vi "Set External Tn.vi"(6 "parseError? T:Yes":bool=TRUE, 8 "error in (no error)":errorcluster, 10 "Tn (3s)":u16=3 min=3 max=9999, 11 "VISA resource name":refnum<visa-resource-name>) -> (0 "error out":errorcluster, 3 "VISA resource name out":refnum<visa-resource-name>)   [LabVIEW 2015, in "JULABO DeviceDriver.lvlib"]
doc: "This VI adjusts the Resetting time <B>Tn</B> (Integral component) in case of external temperature control.\n\nCompensation of the remaining control deviation due to proportional control. An insufficient resetting time may cause instabilities to occur. An excessive resetting time will unnecessarily prolong compensation of the control difference.\nAdjustable range: <B>3 ... 9999</B>\n\nNote:\nThis function is not available for devices which do not have an external sensor plug. For these instruments the VI will return an error (-08 INVALID COMMAND)."
uses:
  JULABO DeviceDriver.lvlib
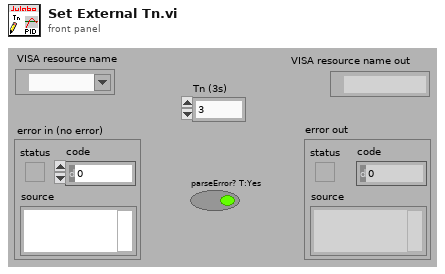
[diagram p1: front panel]
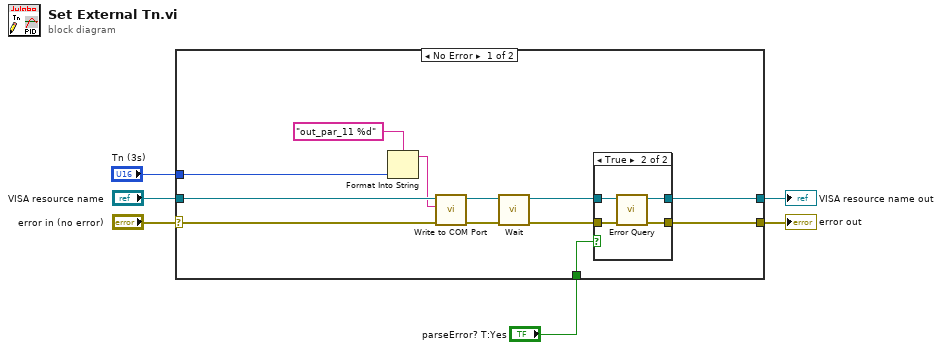
[diagram p0: block diagram]
diagram:
  n1 = case shown="No Error" "error in (no error)" {
    selector: "error in (no error)" -> [w17 w25]
    tunnel: "VISA resource name" -> [w18 w26]
    tunnel: [w15 w25] -> w5
    tunnel: [w14 w26] -> w4
    tunnel: "Tn (3s)" -> [w16 _]
    tunnel: "parseError? T:Yes" -> [w13 _]
    frame No Error {
      n2 = Format Into String(format string="out_par_11 %d", w16) -> (resulting string=w7:string)  [unwired: 2 in, 1 out]
      n3 = call "Write to COM Port.vi"("error in"=w17, "Command (input)"=w7, "VISA resource name in"=w18) -> ("error out"=w11:errorcluster, "VISA resource name out"=w12:refnum<visa-resource-name>)  [unwired: 7 in]
      n4 = call "Wait.vi"("error in"=w11, "VISA resource name in"=w12) -> ("error out"=w9:errorcluster, "VISA resource name out"=w10:refnum<visa-resource-name>)  [unwired: 4 in]
      n5 = case shown="True" w13 {
        tunnel: w10 -> [w20 w24]
        tunnel: w9 -> [w19 w23]
        tunnel: [w20 w22] -> w14
        tunnel: [w19 w21] -> w15
        frame False {
        }
        frame True {
          n6 = call "Error Query.vi"("error in (no error)"=w23, "VISA resource name"=w24) -> ("error out"=w21:errorcluster, "VISA resource name out"=w22:refnum<visa-resource-name>)  [unwired: 6 in, 2 out]
        }
      }
    }
    frame Error {
    }
  }
  "error out" <- w5
  "VISA resource name out" <- w4
